vi "ASAP_SubVI_hexapod.vi"(8 "error in":errorcluster, 9 "Configuration":T1={"Calibration data"={"T1"=[], "K1"=[], "T2"=[], "K2"=[]}, "Block size"=0, "Tasks"={"Analog Input"="", "Counters"=[], "Digital out"=""}, "Light enables"=[], "Demodulator table"=[[[0.7378876894649258, 0.0906125472597644, -0.6039607285908369, -0.9832772754191942, -0.8493406206796001, -0.27206330946071283, 0.4472261971995385, 0.9330716049510009, 0.9318702757288254, 0.44424928196195224, -0.27526191405131173, -0.8510913000722428, -0.9826662061933111, -0.6013068779842613, 0.09392391656034481, 0.7401281017410278, 0.999998617584093], [0.9593453970107514, 0.1749709233028358, -0.8033628936873337, -0.8911502339509838, 0.008923213624955564, 0.8991050710898453, 0.7926080184909147, -0.19251348121496464, -0.9642293036540662, -0.6670744875896746, 0.36954793309667006, 0.9965178637479297, 0.5188245350812338, -0.5339978733406581, -0.9948712031832995, -0.3529066352920418, 0.6802631564678894]], [[0.6950304448649641, 0.029259796336992095, -0.6517839440467688, -0.9926080898406189, -0.8153085153483962, -0.21243243641618328, 0.5013295857114554, 0.9534065050307919, 0.907822232196422, 0.3883709446578477, -0.3338030496133024, -0.8817378051772073, -0.969421151739755, -0.5510839461787943, 0.15490925101319897, 0.7800425818962478, 0.9980075966531081], [0.9381204165433596, 0.10815294018097958, -0.8417045890860233, -0.8585129793585211, 0.07636026142185437, 0.9265863741042095, 0.749669912334455, -0.25827310590600655, -0.979914371470141, -0.615297735575794, 0.43139076953297817, 0.9998725601934042, 0.45997233240039587, -0.5898179378997009, -0.9857812880942376, -0.2889831231211053, 0.728159563799897]], [[-0.6523106754624476, 0.028565353817145308, 0.6945307778513148, 0.9979635224154992, 0.7804771064006715, 0.15559556021784737, -0.5505040934388046, -0.969250428253351, -0.8820653255595329, -0.33445785406592654, 0.38773065238112236, 0.9075306732447919, 0.953615867977217, 0.5019305868317728, -0.2117535089882616, -0.814906049621952, -0.9926921657471056], [-0.8972537749411549, -0.004712231334943897, 0.8930529304466017, 0.800848121012319, -0.17911548107307929, -0.9605254010675951, -0.6771705448338604, 0.3568436305984995, 0.9952883311784719, 0.5304327379276333, -0.5224198982706508, -0.9961579108878458, -0.3656316803152294, 0.6702057828807996, 0.9631045277016598, 0.18837947435655572, -0.7951686133781816]], [[-0.6100621017406637, 0.08296383725289572, 0.7326841328141306, 0.9999563780585607, 0.7452692276197674, 0.10156483182376178, -0.5951545948322141, -0.9812139372354715, -0.8550971038041967, -0.28263483236625087, 0.43735778093254624, 0.9290574326162326, 0.9358056736945096, 0.4540800426756246, -0.2646672723560626, -0.8452629914108203, -0.9846465037423504], [-0.8635658054477633, 0.06644929359614622, 0.9228038031878806, 0.756208806278458, -0.24866126331928293, -0.9778845315929664, -0.6231000231838354, 0.42240537195639455, 0.9996645751178765, 0.468772316125792, -0.5817649722709365, -0.9874022405026531, -0.2984811300725095, 0.7213132642049666, 0.9415151068455686, 0.1180255271232651, -0.8362980980464019]], [[0.5777399532793561, -0.12292948264806108, -0.7594319210118347, -0.9995244406514613, -0.717883028231008, -0.0615194781167083, 0.6269561424089901, 0.9881718380097269, 0.8335794576620439, 0.24387346683869626, -0.4731301243274189, -0.9431682286060581, -0.9208893384307617, -0.41792263714147493, 0.3031922273189156, 0.866046156382817, 0.9768394372642432], [0.817447755955057, -0.151248697507681, -0.9522824474358904, -0.6976889272021819, 0.3303090169266952, 0.992151723408322, 0.5541711388190733, -0.49812105893626973, -0.9982344623949164, -0.391781716958503, 0.6489701857141323, 0.9703235240149266, 0.21605063861728646, -0.777719411171446, -0.9093693817994032, -0.03296221490214164, 0.8799843348529361]], [[0.5316898836029471, -0.17765562828651216, -0.7942680705992896, -0.996286745386534, -0.6782615072995046, -0.006195858817183757, 0.6691039174680259, 0.9951433819294784, 0.8017357488499911, 0.18983635337997448, -0.5211542329290844, -0.9601116041437467, -0.8979078410494362, -0.36701219861201956, 0.3554572660433528, 0.8923843772058451, 0.9635027586436964], [0.7637113666149481, -0.2374642484157223, -0.9754052139040192, -0.632086784107158, 0.41191456619201, 0.9992990270168236, 0.4789372442711362, -0.5723376274536974, -0.9891629102916494, -0.3094780710033723, 0.7132704172557737, 0.9453420370266403, 0.12947999320562298, -0.8299136384717769, -0.8693286745034909, 0.05492737046661055, 0.9182951461013225]], [[-0.46766510452523, 0.24987476117295926, 0.8369844579156289, 0.9872031947765392, 0.6221194701815425, -0.06769952269503568, -0.7221805721079696, -0.9996962425675782, -0.7553883034308853, -0.11678114183164054, 0.5827836930773002, 0.9781458338214649, 0.862933293995299, 0.2972849646367805, -0.42354081435088226, -0.9232858418611823, -0.9410921262071124], [-0.6914685935131194, 0.33845772670298097, 0.9931957747140229, 0.5469531764674864, -0.5055997555832784, -0.9976835839369067, -0.38381192499528316, 0.6555241911872554, 0.9681964752983884, 0.20760041874903146, -0.7831255366749603, -0.9057385969172634, -0.024319329231539785, 0.8840584812667538, 0.8124368769318331, -0.15978992587511148, -0.9548858745902877]], [[-0.41626060082542315, 0.3049343375163701, 0.8669589900081666, 0.9764465114449328, 0.5762463682854527, -0.12474410208699359, -0.7606203759113978, -0.9994663787495118, -0.7166087568048619, -0.05969414412489584, 0.6283797471765561, 0.9884506172535718, 0.8325678935887533, 0.24209957785384775, -0.47474039981005334, -0.9437743555029069, -0.9201749293116044], [-0.631082800787636, 0.4130942080023554, 0.9993466668991985, 0.47780007230646987, -0.5733990296596044, -0.988971953675139, -0.3082464354209303, 0.71417743507813, 0.9449189867097926, 0.12819583587797975, -0.8306353845064933, -0.8686879369574549, 0.05622031910183376, 0.9188070421528223, 0.7628747613883726, -0.23872195854347844, -0.9756898279662225]]]}, 10 "ADC data":dbl[][](array[numeric])=[[0.4233890953707781, 0.059737563753272625, -0.34526321832859963, -0.4370842281402643, -0.1850326932502861, 0.11627349522930426, 0.3480982972524768, 0.14520556157669487, -0.01859340351497344, -0.04275678381581041, 0.0034736843764850063, 0.02845318126523978, -0.05997519222712916, -0.31180249886316935, -0.1913055722069559, 0.09030184950540061, 0.360436060764886], [0.6090161583111819, 0.023732520276295323, -0.5218643351088168, -0.6243751263951983, -0.2834785113270817, 0.15024627064329113, 0.4894786524267905, 0.24355543536140833, 0.052680574834113765, 0.0051379172996168666, -0.03373152132429563, -0.04606924715825583, -0.18644089055291246, -0.46828867250845085, -0.19741842890272493, 0.2275371695300576, 0.5495514119082466], [-0.3627056826684615, 0.03133358461652651, 0.3305597941044889, 0.369221317860794, 0.17977042772246973, -0.09143559265147504, -0.2909675650457234, -0.16731821192728233, -0.07733762070534453, -0.03201928179911879, 0.04986418022173536, 0.07868421992524977, 0.1690489172928197, 0.28346509297598055, 0.06458624334066014, -0.19497008575623961, -0.34731150756447954], [-0.6450181281783133, 0.10571201219829456, 0.611512527243948, 0.6368442793097259, 0.1730174762656655, -0.318779482110553, -0.5129030504438435, -0.1320972814398578, 0.06778669197162364, 0.05759326324280886, -0.031955272844838026, -0.06567198903643284, 0.19175611740982554, 0.49285514286049803, 0.23913881034792678, -0.2701966435703145, -0.6145497005316812], [0.4695717653663261, -0.13065707989874734, -0.48157056823484895, -0.4650882160743811, -0.10884602816301027, 0.2719754623206629, 0.3716696684050737, 0.08025243985520478, -0.05592662595057675, -0.03766807199567128, 0.027317022173162845, 0.04933610623551206, -0.17896784359433077, -0.3703707665898961, -0.16486986906943993, 0.2394908601602379, 0.47870908960882014], [0.668160939441404, -0.26571601376575427, -0.7523298763225447, -0.6841118364455508, -0.18660091297417802, 0.4193565147222573, 0.5509276134493617, 0.16146384928902122, -0.01142440045017552, -0.025378352764062116, -0.011488409406532252, -0.004927491337157158, -0.3586731126626958, -0.5398829220356592, -0.15688475099700663, 0.4466084441328689, 0.748461004808878], [-0.3118825101365961, 0.1851791900696957, 0.4070827491012809, 0.3491544481283409, 0.12969938150207558, -0.21727721323812305, -0.2918476889082694, -0.1374740339016221, -0.07074469855287382, -0.0026391711111129917, 0.06805873010744334, 0.08567720073080362, 0.2530927857458196, 0.2521806565553053, -0.009680156386373016, -0.29677638264989614, -0.4047596372992107], [-0.6122773710321248, 0.443872048993655, 0.8820654900364707, 0.6474378529873531, 0.013395073062435703, -0.6203265386424837, -0.5113668303400581, -0.011152362385570862, 0.1554790069238322, 0.035622185214427414, -0.09994878350250055, -0.1158550087471243, 0.43435067511840836, 0.58534866769129, 0.18177070962625866, -0.5484281507089904, -0.8615301809255184], [-0.06624806961243182, -0.05802291916164041, -0.042420736809552224, -0.03131518330175245, -0.031459203448991, -0.04258075919349681, -0.051510008186773336, -0.051558014901649865, -0.04872561872163144, -0.04810153142705679, -0.04982977316526523, -0.05176604399943352, -0.044020960648023424, -0.03389154370964889, -0.03109115196155207, -0.04093252863778666, -0.05603864161838519], [-0.022401936357063147, -0.022561958744878777, -0.022497949789757297, -0.022241913969207668, -0.022017882626142776, -0.022001880387349414, -0.022113896058894494, -0.02216190277526494, -0.022225911730419923, -0.022241913969207668, -0.022321925163140396, -0.022481947550975934, -0.02243394083462946, -0.022225911730419923, -0.021953873670966927, -0.021873862476988058, -0.022113896058894494], [-0.04461304346772397, -0.04464504794445658, -0.04464504794445658, -0.04464504794445658, -0.04462904570609038, -0.04462904570609038, -0.04462904570609038, -0.04461304346772397, -0.04461304346772397, -0.04462904570609038, -0.04459704122935736, -0.04461304346772397, -0.04464504794445658, -0.044565036752623535, -0.04461304346772397, -0.044565036752623535, -0.04458103899099055], [-0.044565036752623535, -0.044565036752623535, -0.044533032275888895, -0.044533032275888895, -0.04454903451425632, -0.044565036752623535, -0.04454903451425632, -0.04459704122935736, -0.04451703003752128, -0.044533032275888895, -0.044533032275888895, -0.044565036752623535, -0.04459704122935736, -0.04462904570609038, -0.04461304346772397, -0.04461304346772397, -0.04461304346772397]], 11 "timestamp":cluster{"t0":timestamp, "dt":dbl}) -> (0 "error out":errorcluster, 1 "raw output":dbl[][](array[numeric]), 2 "Match error":waveform(dbl)[](array[waveform]), 4 "XYZ out":T3(array[cluster]), 5 "Diagnostics":cluster{"Valid position":bool, "Message":string})   [LabVIEW 2011]
uses:
  asap/labview/initialization/configuration.ctl
  <vilib>/Analysis/Matrix/Datatypes/RealMatrix.ctl
  <vilib>/Analysis/Matrix/NI_Matrix.lvlib
panel:
  in  "display channel":i32
  in  "display freq":i32
  out "Waveform Graph":waveform(sgl)(graph)
  in  "Use LUT":bool
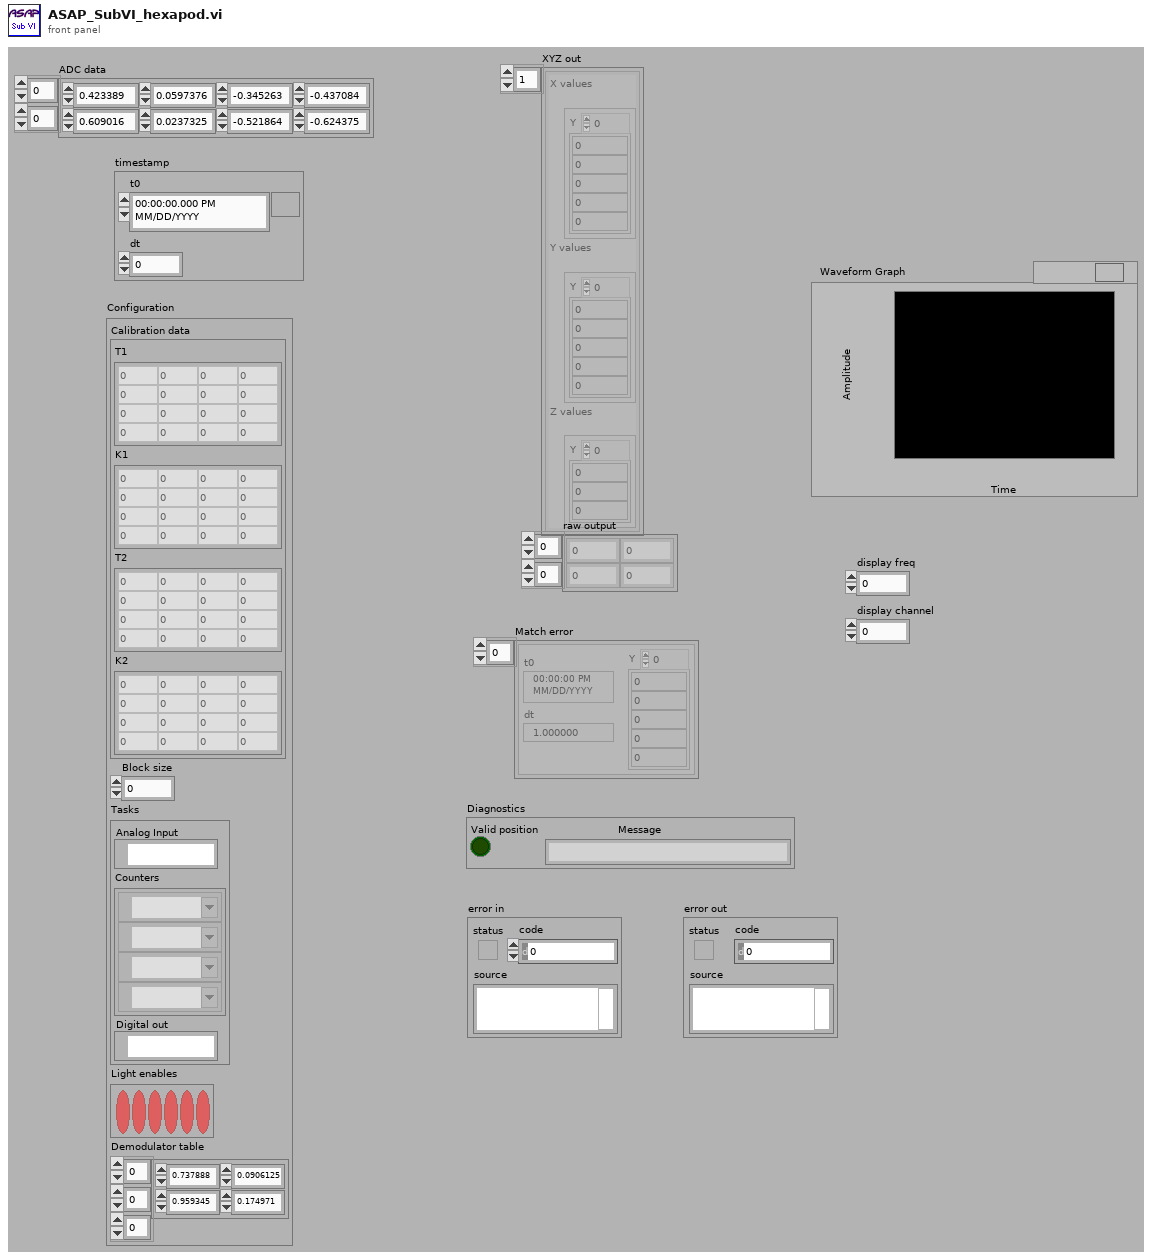
[diagram p1: front panel]
types:
  T1 = typedef "configuration.ctl" = cluster{"Calibration data":cluster{"T1":T2, "K1":T2, "T2":T2, "K2":T2}, "Block size":i32, "Tasks":cluster{"Analog Input":refnum<k21>, "Counters":refnum<k21>[], "Digital out":refnum<k21>}, "Light enables":bool[], "Demodulator table":dbl[][][]}
  T2 = typedef "NI_Matrix.lvlib/RealMatrix.ctl" = dbl[][]
  T3 = cluster{"X values":waveform(dbl), "Y values":waveform(dbl), "Z values":waveform(dbl)}[]
  T4 = cluster{"X values":waveform(sgl), "Y values":waveform(sgl), "Z values":waveform(sgl)}[]
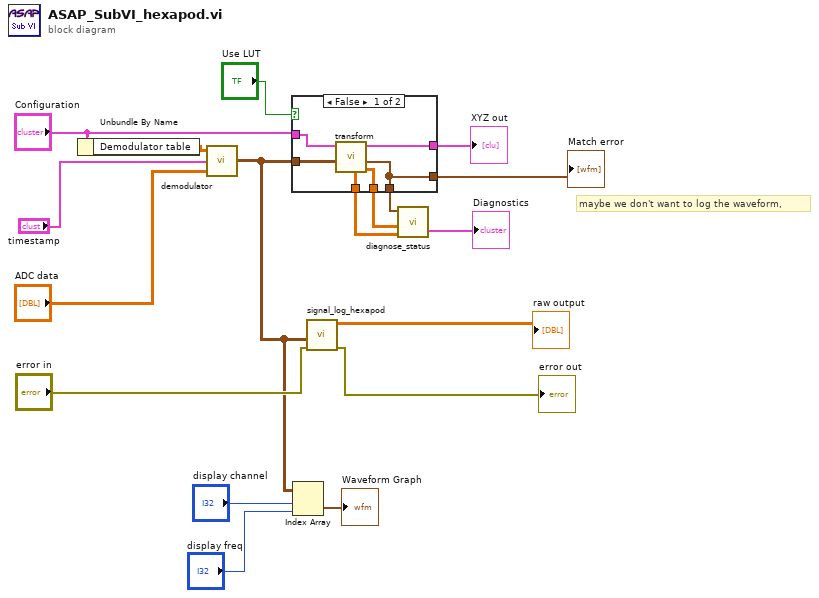
[diagram p0: block diagram]
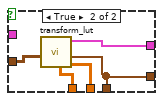
[diagram p2: hidden frame]
diagram:
  # "maybe we don't want to log the waveform,"
  n1 = Unbundle By Name("Configuration") -> ("Demodulator table"=w1:dbl[][][])
  n2 = call "demodulator.vi"("ADC data"="ADC data", "timestamp"="timestamp", "Demodulator table"=w1) -> ("Demodulated signals"=w6:waveform(sgl)[][])
  n3 = case shown="False" "Use LUT" {
    tunnel: w6 -> [w24 w25]
    tunnel: [w23 w28] -> w18
    tunnel: [w22 w29] -> w16
    tunnel: [w20 w26] -> w15
    tunnel: [w21 w27] -> w14
    tunnel: "Configuration" -> [w19 _]
    tunnel: [w20 w26] -> w8
    frame False {
      n4 = call "transform.vi"("Demodulated signals"=w24, "Configuration"=w19) -> ("Sum amplitudes"=w23:sgl[][], "Match error"=w20:waveform(sgl)[], "XYZ out"=w22:T4, "Axis positions"=w21:sgl[][])  [unwired: 6 in]
    }
    frame True {
      n5 = call "transform_lut.vi"("Demodulated signals"=w25) -> ("Sum amplitudes"=w28:sgl[][], "Match error"=w26:waveform(sgl)[], "XYZ out"=w29:T4, "Axis positions"=w27:sgl[][])  [unwired: 7 in]
    }
  }
  "XYZ out" <- w16
  "Match error" <- w8
  n6 = Index Array(array=w6, index (row)="display channel", index (col)="display freq") -> (element=→"Waveform Graph":waveform(sgl))
  n7 = call "signal_log_hexapod.vi"("error in"="error in", "Demodulated signals"=w6) -> ("error out"=→"error out":errorcluster, "raw output"=→"raw output":dbl[][])  [unwired: 8 in]
  n8 = call "diagnose_status.vi"("Match error"=w15, "Sum amplitudes"=w18, "Axis positions"=w14) -> ("Status"=→"Diagnostics":cluster{"Valid position":bool, "Message":string})  [unwired: 3 in]
